vi "MXAQUIS.vi"() -> ()   [LabVIEW 2018]
uses:
  <vilib>/DAQmx/create/channels.llb/DAQmx Create Channel (AI-Voltage-Basic).vi
  <vilib>/DAQmx/configure/timing.llb/DAQmx Timing (Sample Clock).vi
  <vilib>/DAQmx/read.llb/DAQmx Read (Analog DBL 1Chan 1Samp).vi
panel:
  in  "sample mode":i32(ring)=10178 items=["Finite Samples"=10178, "Continuous Samples"=10123, "Hardware Timed Single Point"=12522]
  in  "Durata [s]":dbl=1000.0 format="%0.2f"
  in  "rate":dbl=1000.0 format="%0.2f"
  in  "canale":tag
  in  "input terminal configuration":i32(ring)=-1 items=["Default"=-1, "RSE"=10083, "NRSE"=10078, "Differential"=10106, "Pseudodifferential"=12529]
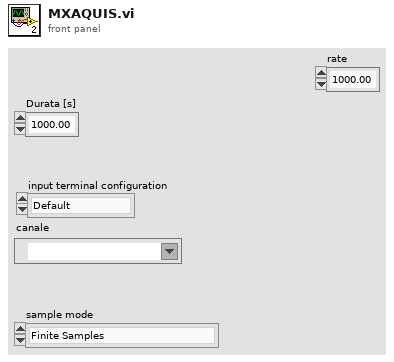
[diagram p1: front panel]
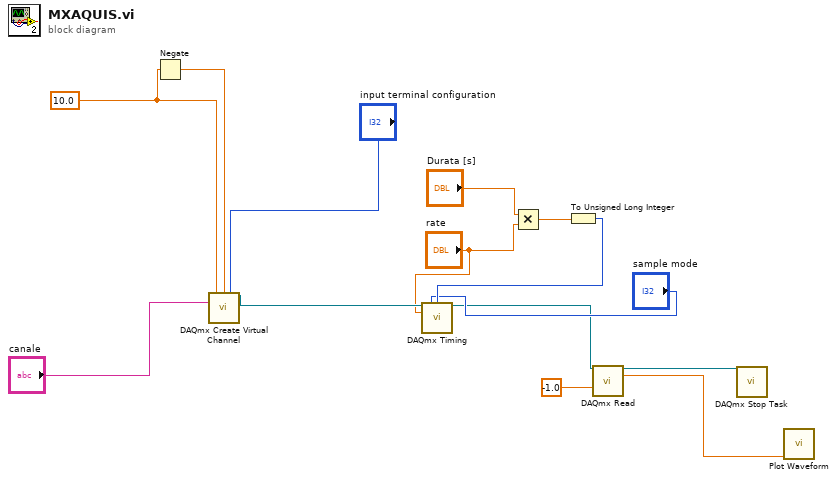
[diagram p0: block diagram]
diagram:
  w12 = 10.0 items=["10"=10.0, "5"=5.0, "0.5  or 1"=0.5, "0.05 or 0.2"=0.05] ("Fondo Scala")
  n1 = Negate(x=w12) -> (-x=w11:dbl)
  n2 = call-poly <vilib>:"DAQmx Create Virtual Channel.vi"("maximum value"=w12, "minimum value"=w11, "input terminal configuration"="input terminal configuration", "physical channels"="canale") -> ("task out"=w10:refnum<k21>)  [unwired: 10 in, 1 out]
  n3 = Multiply(x="Durata [s]", y="rate") -> (x*y=w7:dbl)
  n4 = To Unsigned Long Integer(number=w7) -> (unsigned 32bit integer=w6:u32)
  n5 = call-poly <vilib>:"DAQmx Timing.vi"("task/channels in"=w10, "sample mode"="sample mode", "samples per channel"=w6, "rate"="rate") -> ("task out"=w4:refnum<k21>)  [unwired: 10 in, 1 out]
  n6 = call-poly <vilib>:"DAQmx Read.vi"("task/channels in"=w4, "timeout"=-1.0) -> ("task out"=w3:refnum<k21>, "data"=w1:dbl)  [unwired: 11 in, 1 out]
  n7 = call <vilib>:"DAQmx Stop Task.vi"("task/channels in"=w3) -> ()  [unwired: 13 in, 2 out]
  n8 = call <vilib>:"Plot Waveform.vi"("waveform data"=w1) -> ()  [unwired: 10 in, 1 out]
